vi "Yields.vi"(7 "Station":i32, 8 "Control":T1, 9 "UUT State":string, 10 "General.Sequence Path":path, 11 "Socket":i32) -> (0 "error out":errorcluster)   [LabVIEW 2025, in "Test Unit.lvlib"]
uses:
  Test Unit.lvlib
panel:
  in  "error in (no error)":errorcluster
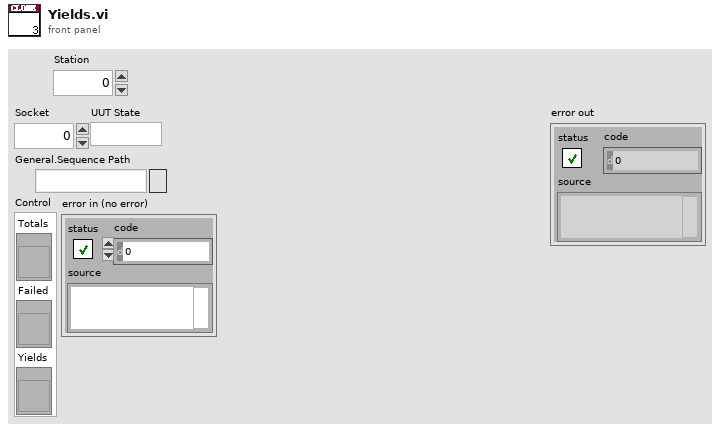
[diagram p1: front panel]
types:
  T1 = cluster{"Totals":refnum<vi>, "Failed":refnum<vi>, "Yields":refnum<vi>}
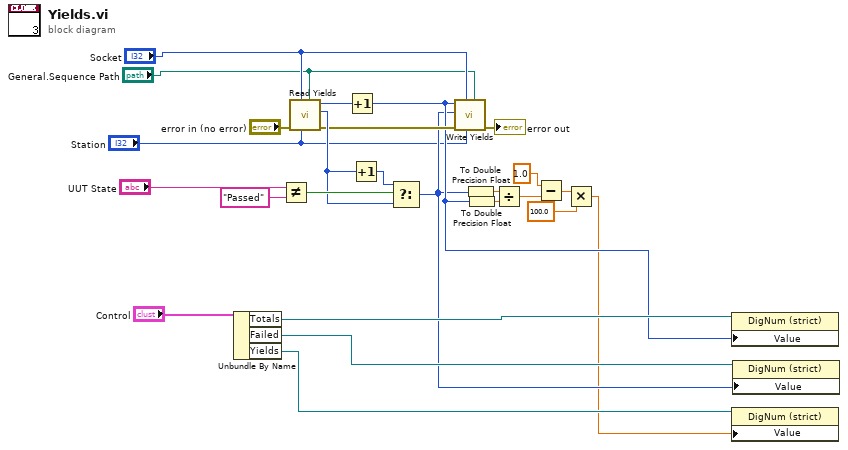
[diagram p0: block diagram]
diagram:
  n1 = Unbundle By Name("Control") -> ("Totals"=w10:refnum<vi>, "Failed"=w9:refnum<vi>, "Yields"=w8:refnum<vi>)
  n2 = Not Equal?(x="UUT State", y="Passed") -> (x != y?=w23:bool)
  n3 = call "Read Yields.vi"("General.Sequence Path"="General.Sequence Path", "Station"="Station", "Socket"="Socket", "error in (no error)"="error in (no error)") -> ("error out"=w7:errorcluster, "Failed"=w21:i32, "Totals"=w25:i32)  [unwired: 5 in]
  n4 = Increment(x=w25) -> (x+1=w4:i32)
  n5 = Increment(x=w21) -> (x+1=w22:i32)
  n6 = Select(t=w22, s=w23, f=w21) -> (s? t:f=w3:i32)
  n7 = call "Write Yields.vi"("General.Sequence Path"="General.Sequence Path", "Station"="Station", "Socket"="Socket", "error in (no error)"=w7, "Failed"=w3, "Totals"=w4) -> ("error out"=→"error out":errorcluster)  [unwired: 5 in]
  n8 = To Double Precision Float(number=w3) -> (double precision float=w20:dbl)
  n9 = To Double Precision Float(number=w4) -> (double precision float=w19:dbl)
  n10 = Divide(x=w20, y=w19) -> (x/y=w18:dbl)
  n11 = Subtract(x=1.0, y=w18) -> (x-y=w16:dbl)
  n12 = Multiply(x=w16, y=100.0) -> (x*y=w2:dbl)
  n13 = property class="DigNum (strict)"(reference=w10, "Value"=w4) -> ()  [unwired: 1 in, 2 out]
  n14 = property class="DigNum (strict)"(reference=w8, "Value"=w2) -> ()  [unwired: 1 in, 2 out]
  n15 = property class="DigNum (strict)"(reference=w9, "Value"=w3) -> ()  [unwired: 1 in, 2 out]
